vi "PVCAM_StopCont.vi"(8 "error in (no error)":errorcluster, 10 "cam_state":T1(ring)=enum."CCS_HALT", 11 "hCam":i16) -> (0 "error out":errorcluster, 2 "return":i16)   [LabVIEW 2021]
uses:
  pvcam64.dll
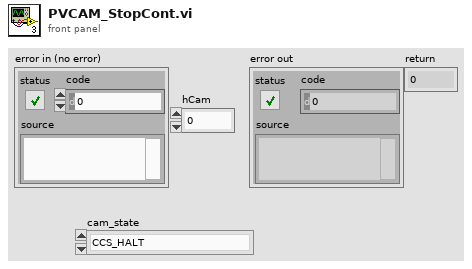
[diagram p1: front panel]
types:
  T1 = enum16{"CCS_NO_CHANGE", "CCS_HALT", "CCS_HALT_CLOSE_SHTR", "CCS_CLEAR", "CCS_CLEAR_CLOSE_SHTR", "CCS_OPEN_SHTR", "CCS_CLEAR_OPEN_SHTR"}
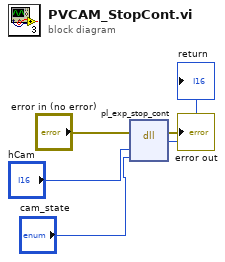
[diagram p0: block diagram]
diagram:
  n1 = dll-call lib="pvcam64.dll" fn="pl_exp_stop_cont"(error in="error in (no error)", "hCam"="hCam", "cam_state"="cam_state") -> (error out=→"error out":errorcluster, "return type"=→"return":i16)  [unwired: 4 in, 1 out]
